vi "Register gRPC Parameters.vi"(8 "error in (no error)":errorcluster, 11 "OOP Server in":refnum<class "TestDataMarshal.lvclass">) -> (0 "error out":errorcluster, 3 "OOP Server out":refnum<class "TestDataMarshal.lvclass">)   [LabVIEW 2019, in "TestDataMarshal.lvlib" / "TestDataMarshal.lvclass"]
uses:
  TestDataMarshal.lvclass
  TestDataMarshal.lvclass/TestDataMarshal.ctl
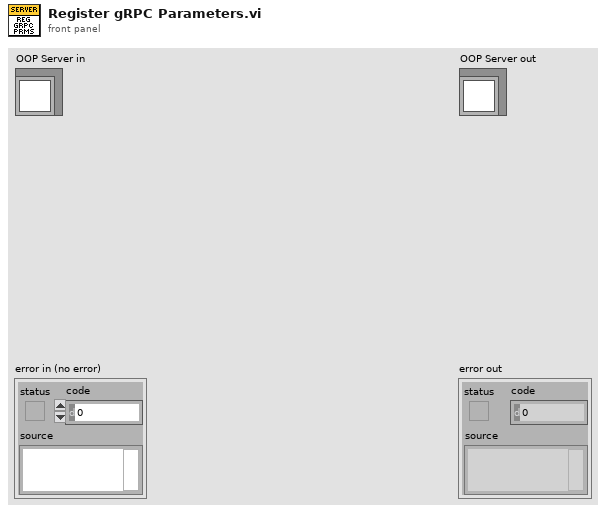
[diagram p1: front panel]
types:
  T1 = typedef "TestDataMarshal.lvlib/gprc-lvsupport.lvlib/grpcId.ctl" = u64
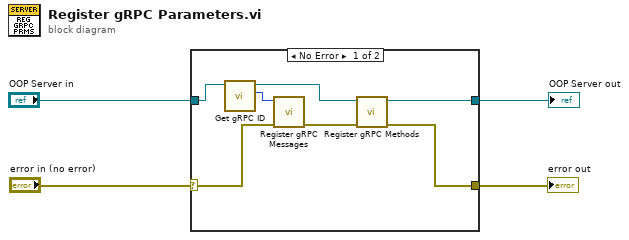
[diagram p0: block diagram]
diagram:
  n1 = case shown="No Error" "error in (no error)" {
    selector: "error in (no error)" -> [w11 w13]
    tunnel: [w9 w13] -> w3
    tunnel: [w5 w12] -> w1
    tunnel: "OOP Server in" -> [w8 w12]
    frame No Error {
      n2 = call "Get gRPC ID.vi"("OOP Server in"=w8) -> ("gRPC ID"=w7:T1, "OOP Server out"=w6:refnum<class "TestDataMarshal.lvclass">)  [unwired: 9 in]
      n3 = call "Register gRPC Messages.vi"("error in (no error)"=w11, "gRPC ID"=w7) -> ("error out"=w10:errorcluster)  [unwired: 8 in, 1 out]
      n4 = call "Register gRPC Methods.vi"("error in (no error)"=w10, "Template Server in"=w6) -> ("error out"=w9:errorcluster, "Template Server out"=w5:refnum<class "TestDataMarshal.lvclass">)  [unwired: 8 in]
    }
    frame Error {
    }
  }
  "error out" <- w3
  "OOP Server out" <- w1
